vi "Write to VI Description (Recursive).vi"(8 "error in (no error)":errorcluster, 10 "License Text to Add":string, 11 "ProjectItem in":refnum<vi>) -> (0 "error out":errorcluster)   [LabVIEW 2012, in "Add License to VI Documentation.lvlib"]
uses:
  Add License to VI Documentation.lvlib
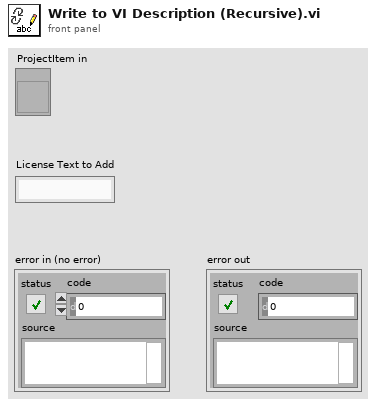
[diagram p1: front panel]
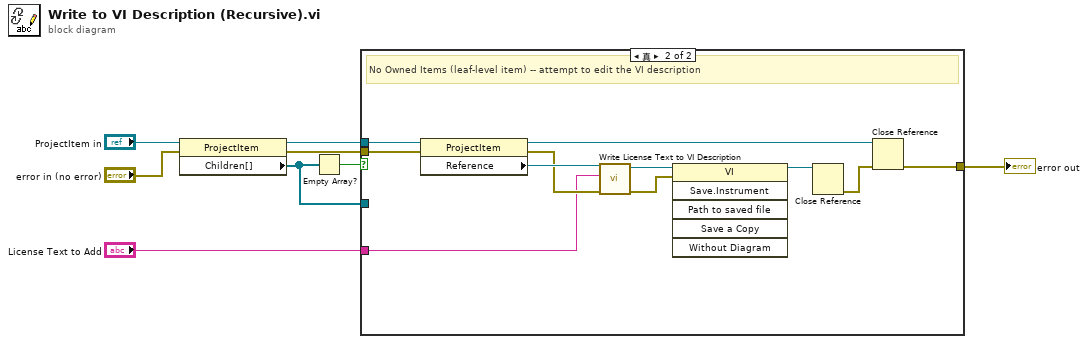
[diagram p0: block diagram]
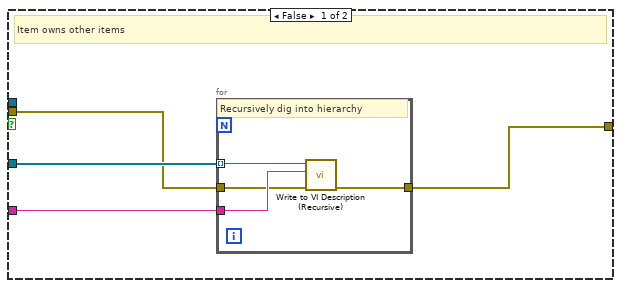
[diagram p2: hidden frame]
diagram:
  n1 = property on="Property Node" class="ProjectItem"(reference="ProjectItem in", error in="error in (no error)") -> (reference out=w6:refnum<vi>, error out=w5:errorcluster, "Children[]"=w3:refnum<vi>[])
  n2 = Empty Array?(array=w3) -> (empty?=w4:bool)
  n3 = case shown="真" w4 {
    tunnel: w6 -> [_ w27]
    tunnel: w5 -> [w9 w17]
    tunnel: w3 -> [w12 _]
    tunnel: [w11 w25] -> w2
    tunnel: "License Text to Add" -> [w10 w19]
    frame False {
      # "Item owns other items"
      n4 = for {
        tunnel: w12 -> [w16] mode=indexing
        tunnel: [w15] -> w11
        tunnel: w10 -> [w14]
        tunnel: w9 -> [w13]
        # "Recursively dig into hierarchy"
        n5 = call "Write to VI Description (Recursive).vi"("error in (no error)"=w13, "License Text to Add"=w14, "ProjectItem in"=w16) -> ("error out"=w15:errorcluster)  [unwired: 8 in]
      }
    }
    frame True {
      # "No Owned Items (leaf-level item) -- attempt to edit the VI description"
      n6 = property on="Property Node" class="ProjectItem"(reference=w27, error in=w17) -> (reference out=w26:refnum<vi>, error out=w22:errorcluster, "Reference"=w24:refnum<vi>)
      n7 = call "Write License Text to VI Description.vi"("error in (no error)"=w22, "String"=w19, "VI in"=w24) -> ("error out"=w21:errorcluster, "VI out"=w23:refnum<vi>)  [unwired: 7 in]
      n8 = invoke class="VI" method="Save.Instrument"(reference=w23, error in=w21) -> (reference out=w20:refnum<vi>)  [unwired: 4 in, 5 out]
      n9 = Close Reference(reference=w20) -> (error out=w18:errorcluster)  [unwired: 1 in]
      n10 = Close Reference(reference=w26, error in (no error)=w18) -> (error out=w25:errorcluster)
    }
  }
  "error out" <- w2
